vi "Close Pipe.vi"   [LabVIEW 2016, in "Linux RT IPC.Pipes.lvlib"]
doc: "This VI closes the endpoint, preventing the endpoint from reading from or writing to the pipe. This does not remove the pipe from the filesystem, so other endpoints can continue to use the pipe."
uses:
  Linux RT IPC.Pipes.lvlib
  Classes/Unix Pipe Writer/Unix Pipe Writer.lvclass
  Classes/Unix Pipe Reader/Unix Pipe Reader.lvclass
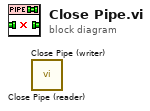
[diagram p0: block diagram]
diagram:
  n1 = call "Close Pipe (reader).vi"() -> ()  [unwired: 10 in, 2 out]
  n2 = call "Close Pipe (writer).vi"() -> ()  [unwired: 10 in, 2 out]
